vi "State_machine.vi"() -> ()   [LabVIEW 2022 SP3]
panel:
  out "Actual state":enum16{"Items", "Wait", "Measure", "End", ""}(ring)
  in  "Enum":enum16{"Items", "Wait", "Measure", "End", ""}(ring)
  in  "Stop Button":bool
  in  "Start Meassuring":bool
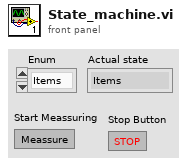
[diagram p1: front panel]
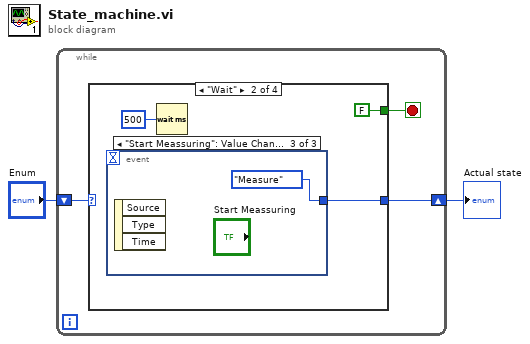
[diagram p0: block diagram]
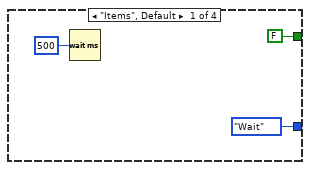
[diagram p2: hidden frame]
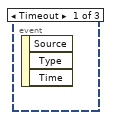
[diagram p3: hidden frame]
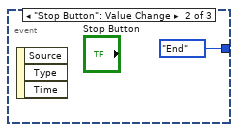
[diagram p4: hidden frame]
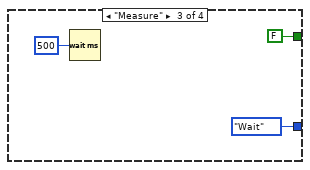
[diagram p5: hidden frame]
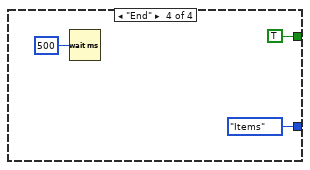
[diagram p6: hidden frame]
diagram:
  n1 = while {
    shift-right: [w4] -> w1
    shift-left: "Enum" -> [w5]
    stop <- w3 stop-if-true
    n2 = case shown="\"Wait\"" w5 {
      tunnel: [enum16{"Items", "Wait", "Measure", "End"}."Wait" ("Enum 2") w9 enum16{"Items", "Wait", "Measure", "End"}."Wait" ("Enum 2") enum16{"Items", "Wait", "Measure", "End"}."Items" ("Enum 2")] -> w4
      tunnel: [FALSE FALSE FALSE TRUE] -> w3
      frame "Items", Default {
        n3 = Wait (ms)(milliseconds to wait=u32 500) -> ()  [unwired: 1 out]
      }
      frame "Wait" {
        n4 = event shown="[2] \"Start Meassuring\": Value Change" {
          selector: _ -> [_ _ _]
          dyn-events: _ -> [_ _ _]
          timeout: _ -> [_ _ _]
          tunnel: [_ enum16{"Items", "Wait", "Measure", "End"}."End" ("Enum 2") enum16{"Items", "Wait", "Measure", "End"}."Measure" ("Enum 2")] -> w9
          event Timeout {
            n5 = event-data() -> ()  [unwired: 1 in, 3 out]
          }
          event "Stop Button": Value Change {
            n6 = event-data() -> ()  [unwired: 1 in, 3 out]
          }
          event "Start Meassuring": Value Change {
            n7 = event-data() -> ()  [unwired: 1 in, 3 out]
          }
        }
        n8 = Wait (ms)(milliseconds to wait=u32 500) -> ()  [unwired: 1 out]
      }
      frame "Measure" {
        n9 = Wait (ms)(milliseconds to wait=u32 500) -> ()  [unwired: 1 out]
      }
      frame "End" {
        n10 = Wait (ms)(milliseconds to wait=u32 500) -> ()  [unwired: 1 out]
      }
    }
  }
  "Actual state" <- w1
